vi "Match Window Size.vi"(8 "错误输入（无错误）":errorcluster, 10 "界面单元":refnum<vi>, 11 "VI输入":refnum<vi>) -> (0 "错误输出":errorcluster, 3 "窗口边界":T1)   [LabVIEW 2020]
uses:
  <vilib>/Utility/miscctls.llb/LVRectTypeDef.ctl
  <vilib>/Utility/miscctls.llb/LVPositionTypeDef.ctl
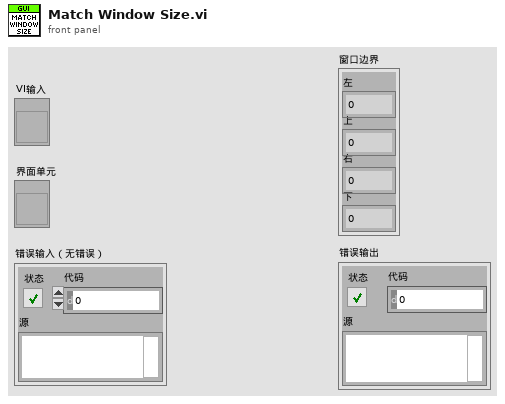
[diagram p1: front panel]
types:
  T1 = typedef "LVRectTypeDef.ctl" = cluster{"Left":i16, "Top":i16, "Right":i16, "Bottom":i16}
  T2 = typedef "LVPositionTypeDef.ctl" = cluster{"Left":i32, "Top":i32}
  T3 = typedef "LVBoundsTypeDef.ctl" = cluster{"Width":u32, "Height":u32}
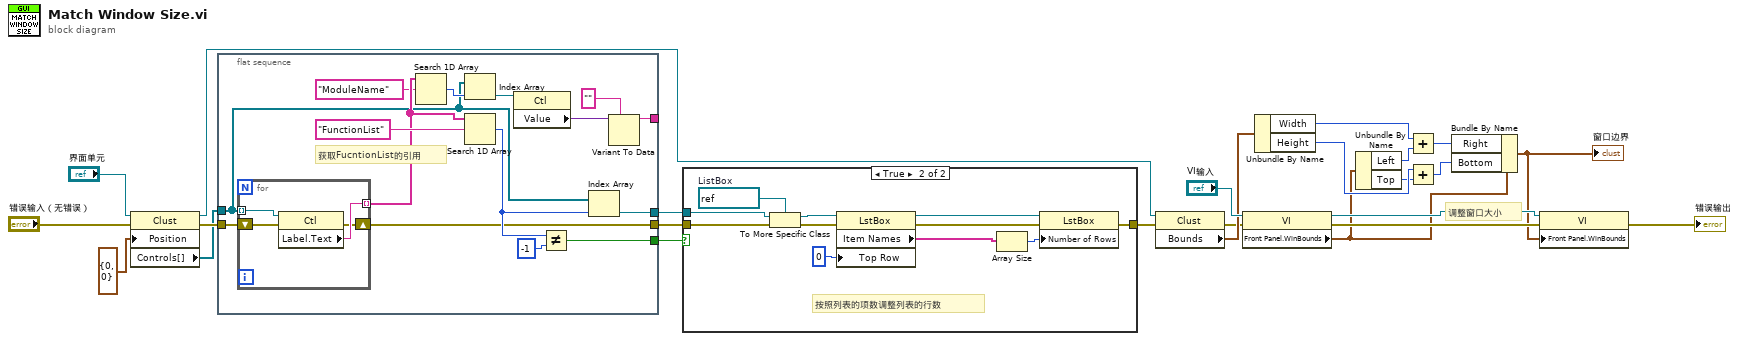
[diagram p0: block diagram]
diagram:
  # "调整窗口大小"
  n1 = property class="Clust"(reference="界面单元", error in="错误输入（无错误）", "Position"=T2 {"Left"=0, "Top"=0} ("位置")) -> (reference out=w7:refnum<vi>, error out=w5:errorcluster, "Controls[]"=w2:refnum<vi>[])
  n2 = flat-sequence {
    tunnel: [w37] -> w11
    tunnel: w2 -> [w29]
    tunnel: [w35] -> w6
    tunnel: w5 -> [w34]
    tunnel: [w33] -> w4
    tunnel: [w25] -> _
    frame #0 {
      # "获取FucntionList的引用"
      n3 = for {
        tunnel: w29 -> [w43] mode=indexing
        tunnel: [w42] -> w32 mode=indexing
        shift-right: [w40] -> w33
        shift-left: w34 -> [w41]
        n4 = property class="Ctl"(reference=w43, error in=w41) -> (error out=w40:errorcluster, "Label.Text"=w42:string)  [unwired: 1 out]
      }
      n5 = Search 1D Array(1D array=w32, element="ModuleName" ("元素")) -> (index of element=w30:i32)  [unwired: 1 in]
      n6 = Index Array(array=w29, index=w30) -> (element=w28:refnum<vi>)
      n7 = Search 1D Array(1D array=w32, element="FunctionList" ("元素")) -> (index of element=w36:i32)  [unwired: 1 in]
      n8 = property class="Ctl"(reference=w28) -> ("Value"=w27:variant)  [unwired: 1 in, 2 out]
      n9 = Not Equal?(x=w36, y=-1) -> (x != y?=w37:bool)
      n10 = Index Array(array=w29, index=w36) -> (element=w35:refnum<vi>)
      n11 = Variant To Data(type="", Variant=w27) -> (data=w25:string)  [unwired: 1 in, 1 out]
    }
  }
  n12 = case shown="True" w11 {
    tunnel: [_ w48] -> w8
    tunnel: w6 -> [_ w47]
    tunnel: w4 -> [_ w44]
    frame False {
    }
    frame True {
      w54 = refnum<vi> refnum  # ListBox
      # "按照列表的项数调整列表的行数"
      n13 = To More Specific Class(target class=w54, reference=w47, error in=w44) -> (specific class reference=w45:refnum<vi>, error out=w53:errorcluster)
      n14 = property class="LstBox"(reference=w45, error in=w53, "Top Row"=0 ("顶行")) -> (reference out=w51:refnum<vi>, error out=w49:errorcluster, "Item Names"=w52:string[])
      n15 = Array Size(array=w52) -> (size(s)=w50:i32)
      n16 = property class="LstBox"(reference=w51, error in=w49, "Number of Rows"=w50) -> (error out=w48:errorcluster)  [unwired: 1 out]
    }
  }
  n17 = property class="Clust"(reference=w7, error in=w8) -> (error out=w9:errorcluster, "Bounds"=w10:T3)  [unwired: 1 out]
  n18 = property class="VI"(reference="VI输入", error in=w9) -> (reference out=w24:refnum<vi>, error out=w23:errorcluster, "Front Panel.WinBounds"=w16:T1)
  n19 = Unbundle By Name(w10) -> ("Width"=w20:u32, "Height"=w19:u32)
  n20 = Unbundle By Name(w16) -> ("Left"=w17:i16, "Top"=w18:i16)
  n21 = Add(x=w20, y=w17) -> (x+y=w21:u32)
  n22 = Add(x=w19, y=w18) -> (x+y=w22:u32)
  n23 = Bundle By Name(cluster=w16, "Right"=w21, "Bottom"=w22) -> (w1:T1)
  "窗口边界" <- w1
  n24 = property class="VI"(reference=w24, error in=w23, "Front Panel.WinBounds"=w1) -> (error out=→"错误输出":errorcluster)  [unwired: 1 out]
